vi "Util_App Config File Path.vi"(11 "Config File Name":string="config.ini") -> (3 "Configuration File Path":path)   [LabVIEW 2023]
doc: "This VI returns a path for an application config file located in the same directory as the top level VI or application."
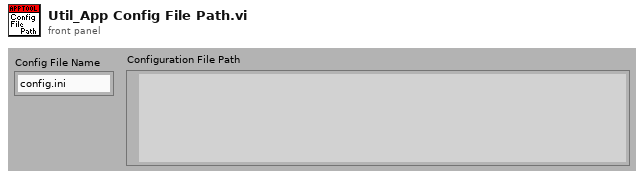
[diagram p1: front panel]
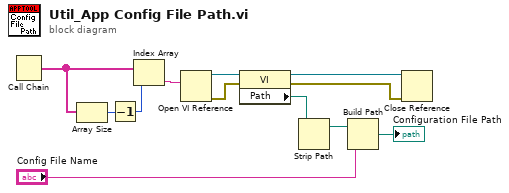
[diagram p0: block diagram]
diagram:
  n1 = Call Chain() -> (call chain=w11:string[])
  n2 = Array Size(array=w11) -> (size(s)=w10:i32)
  n3 = Decrement(x=w10) -> (x-1=w9:i32)
  n4 = Index Array(array=w11, index=w9) -> (element=w8:string)
  n5 = Open VI Reference(vi path=w8) -> (vi reference=w6:refnum<vi>, error out=w7:errorcluster)  [unwired: 1 in, 4 out]
  n6 = property class="VI"(reference=w6, error in=w7) -> (reference out=w5:refnum<vi>, error out=w4:errorcluster, "Path"=w3:path)
  n7 = Strip Path(path=w3) -> (stripped path=w2:path)  [unwired: 1 out]
  n8 = Build Path(base path=w2, name or relative path="Config File Name") -> (appended path=→"Configuration File Path":path)
  n9 = Close Reference(reference=w5, error in (no error)=w4) -> ()  [unwired: 1 out]
